vi "Initialize Analog Edge Trigger.vi"(8 "error in (no error)":errorcluster, 11 "Analog Edge Trigger in":refnum<class "Analog Edge Trigger.lvclass">) -> (0 "error out":errorcluster, 3 "Analog Edge Trigger out":refnum<class "Analog Edge Trigger.lvclass">)   [LabVIEW 2015, in "Analog Edge Trigger.lvclass"]
uses:
  Analog Edge Trigger.lvclass
  Analog Edge Trigger.lvclass/Analog Edge Trigger.ctl
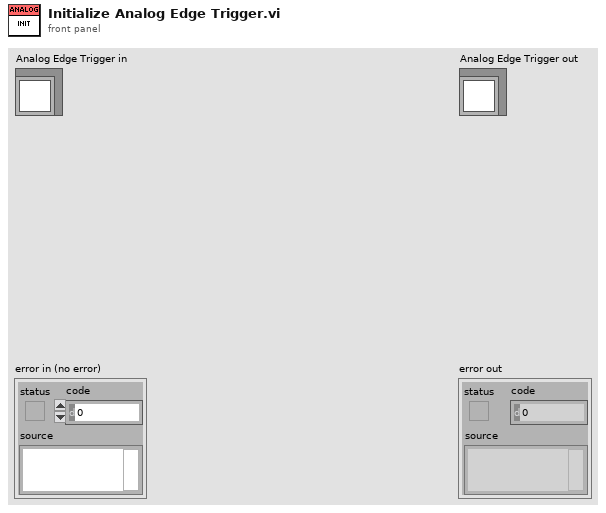
[diagram p1: front panel]
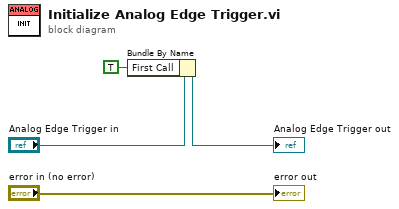
[diagram p0: block diagram]
diagram:
  n1 = Bundle By Name(cluster="Analog Edge Trigger in", "First Call"=TRUE) -> (→"Analog Edge Trigger out":refnum<class "Analog Edge Trigger.lvclass">)
  "error out" <- "error in (no error)"
